vi "getSalveMaster.vi"(11 "direction":T1) -> (2 "Master":i32, 3 "Slave":i32)   [LabVIEW 2011]
uses:
  TapeDrive/Direction_TypDef.ctl
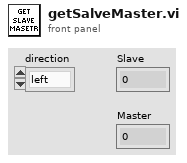
[diagram p1: front panel]
types:
  T1 = typedef "Direction_TypDef.ctl" = enum16{"left", "right"}
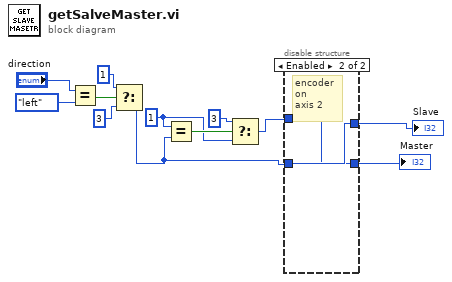
[diagram p0: block diagram]
diagram:
  w10 = 1 ("x")
  n1 = Equal?(x="direction", y=Direction_TypDef."left") -> (x = y?=w8:bool)
  n2 = Select(t=1, s=w8, f=3 ("t")) -> (s? t:f=w2:i32)
  n3 = Equal?(x=w10, y=w2) -> (x = y?=w12:bool)
  n4 = Select(t=3 ("x"), s=w12, f=w10) -> (s? t:f=w4:i32)
  n5 = disable-structure shown="Enabled" {
    disable-tunnel: w4 -> [w14 w15]
    disable-tunnel: [w14 w16] -> w3
    disable-tunnel: w2 -> [w13 w16]
    disable-tunnel: [w13 w15] -> w1
    frame Disabled {
      # "encoder \non \naxis 1"
    }
    frame Enabled {
      # "encoder \non \naxis 2"
    }
  }
  "Slave" <- w3
  "Master" <- w1
